vi "Get WhileLoop LoopTunnels.vi"(8 "error in":errorcluster, 11 "vi path":path=path "C:/Users/lubo/Documents/LabView/LabVIEW-Universal-Transcriptor/Test/Example Test 3.vi") -> (0 "error out":errorcluster, 2 "Tunnels Connected Wires Names":T2(array[cluster]), 3 "LoopTunnels with Terminals array":T3(array[cluster]))   [LabVIEW 2014]
doc: "Return array of clusters contains referencies to LoopTunnel for all WhileLoops. Each row in result array of cluster contain cluster with these items:\n - LoopTunnel ref. array\n - wires labels connected to InsideTerms[]"
uses:
  <vilib>/Utility/traverseref.llb/TRef TravTarget.ctl
  <vilib>/Utility/traverseref.llb/VI Scripting - Traverse.lvlib
panel:
  out "Tunnels Terminals Datatypes[][]":T1(array[cluster])
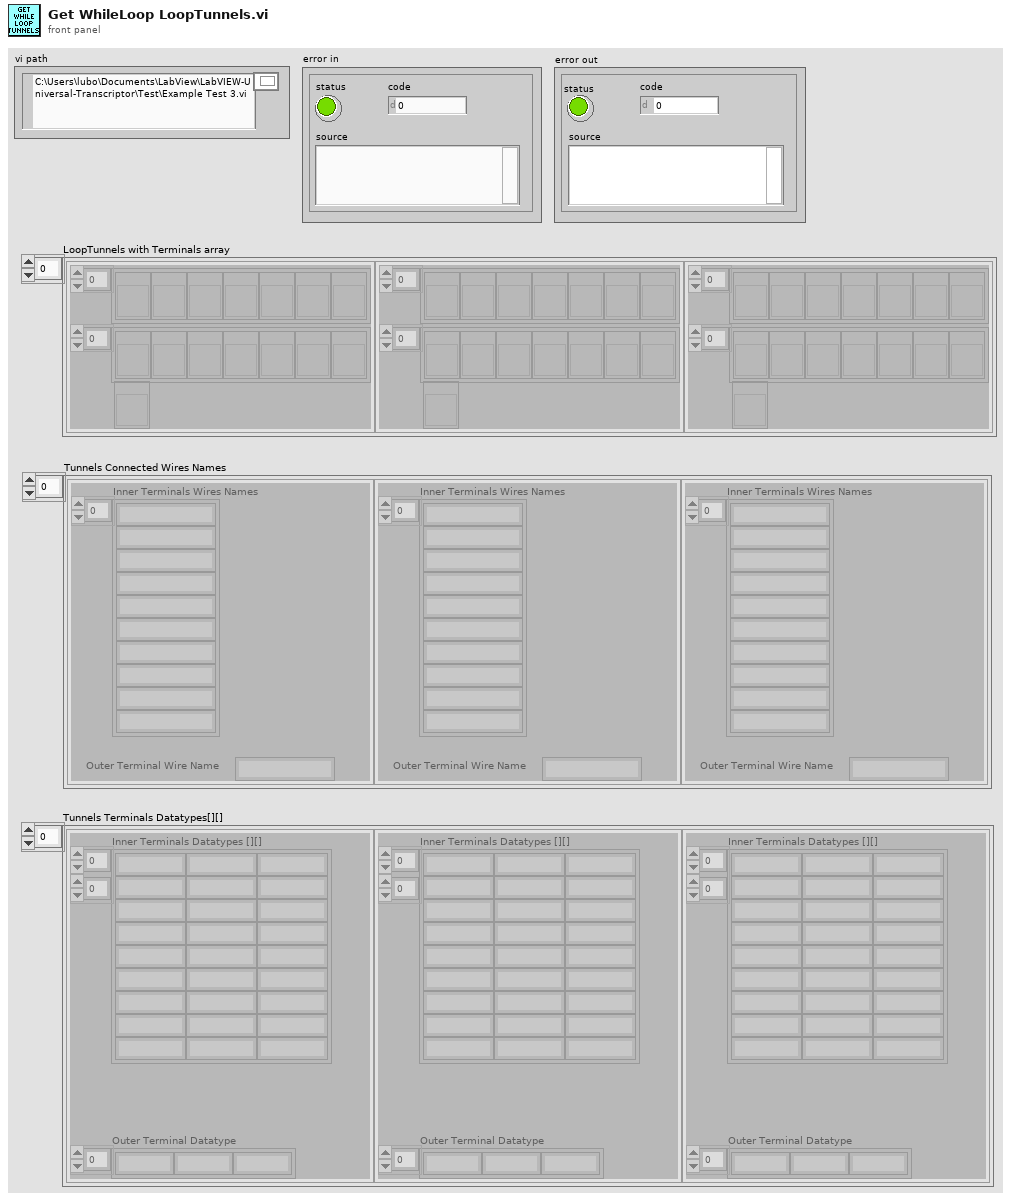
[diagram p1: front panel]
types:
  T1 = cluster{"Inner Terminals Datatypes [][]":string[][], "Outer Terminal Datatype":string[]}[]
  T2 = cluster{"Inner Terminals Wires Names":string[], "Outer Terminal Wire Name":string}[]
  T3 = cluster{refnum<vi>[], refnum<vi>[], refnum<vi>}[]
  T4 = typedef "TRef TravTarget.ctl" = enum16{"FP", "BD", "Other"}
  T5 = cluster{refnum<vi>[], "Inside Terminals[]":refnum<vi>[], "Outside Terminal":refnum<vi>}
  T6 = cluster{refnum<vi>[], "Inside Terminals[]":refnum<vi>[], "Outside Terminal":refnum<vi>}[]
  T7 = cluster{"Inner Terminals Wires Names":string[], "Outer Terminal Wire Name":string}
  T8 = cluster{"Inner Terminals Datatypes [][]":string[][], "Outer Terminal Datatype":string[]}
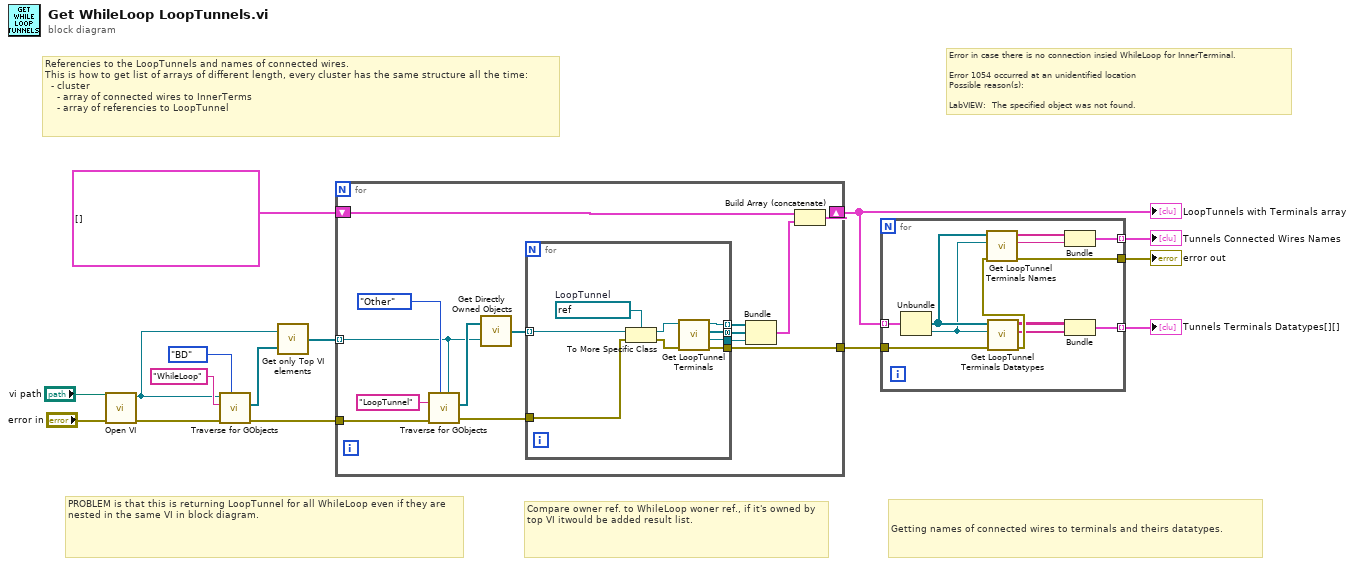
[diagram p0: block diagram]
diagram:
  # "Getting names of connected wires to terminals and theirs datatypes."
  # "Compare owner ref. to WhileLoop woner ref., if it's owned by top VI itwould be added result list."
  # "PROBLEM is that this is returning LoopTunnel for all WhileLoop even if they are nested in the same VI in block diagram."
  # "Error in case there is no connection insied WhileLoop for InnerTerminal.\n\nError 1054 occurred at an unidentified location\nPossible reason(s):\n\nLabVIEW:  The specified object was not found."
  # "Referencies to the LoopTunnels and names of connected wires.\nThis is how to get list of arrays of different length, every cluster has the same structure all the time:\n  - cluster\n    - array of connected wires to InnerTerms\n    - array of referencies to LoopTunnel"
  n1 = call "Open VI.vi"("error in"="error in", "vi path"="vi path") -> ("error out"=w12:errorcluster, "vi reference"=w8:refnum<vi>)  [unwired: 8 in]
  n2 = call <vilib>:"Traverse for GObjects.vi"("Traverse Target"=TRef_TravTarget."BD", "error in (no error)"=w12, "Class Name"="WhileLoop", "VI Refnum"=w8) -> ("error out"=w10:errorcluster, "References"=w7:refnum<vi>[])  [unwired: 4 in, 2 out]
  n3 = call "Get only Top VI elements.vi"("Ref. array in"=w7, "VI ref."=w8) -> ("Ref. array out"=w6:refnum<vi>[])
  n4 = for {
    tunnel: w10 -> [w29]
    tunnel: [w28] -> w4
    shift-right: [w23] -> w5
    shift-left: T3 [] -> [w27]
    tunnel: w6 -> [w20] mode=indexing
    n5 = call <vilib>:"Traverse for GObjects.vi"("Other Refnum"=w20, "Traverse Target"=TRef_TravTarget."Other", "error in (no error)"=w29, "Class Name"="LoopTunnel") -> ("error out"=w25:errorcluster, "References"=w22:refnum<vi>[])  [unwired: 4 in, 2 out]
    n6 = call "Get Directly Owned Objects.vi"("Top Object"=w20, "Nested Objects"=w22) -> ("Directly Owned Objects"=w21:refnum<vi>[])
    n7 = for {
      tunnel: w25 -> [w38]
      tunnel: [w37] -> w28
      tunnel: [w36] -> w19 mode=concatenating
      tunnel: w21 -> [w32] mode=indexing
      tunnel: [w31] -> w18
      tunnel: [w30] -> w17 mode=indexing
      w34 = refnum<vi> refnum  # LoopTunnel
      n8 = To More Specific Class(target class=w34, reference=w32, error in=w38) -> (specific class reference=w35:refnum<vi>, error out=w33:errorcluster)
      n9 = call "Get LoopTunnel Terminals.vi"("error in (no error)"=w33, "LoopTunnel in"=w35) -> ("error out"=w37:errorcluster, "Outside Terminal"=w31:refnum<vi>, "Inside Terminals[]"=w36:refnum<vi>[], "LoopTunnel out"=w30:refnum<vi>)  [unwired: 6 in]
    }
    n10 = Bundle(w17, "Inside Terminals[]"=w19, "Outside Terminal"=w18) -> (w16:T5)  [unwired: 1 in]
    n11 = Build Array (concatenate)(w27, w16) -> (w23:T6)
  }
  "LoopTunnels with Terminals array" <- w5
  n12 = for {
    tunnel: w5 -> [w50] mode=indexing
    tunnel: w4 -> [w45]
    tunnel: [w42] -> w2 mode=indexing
    tunnel: [w43] -> w3
    tunnel: [w41] -> w1 mode=indexing
    n13 = Unbundle(w50) -> (w47:refnum<vi>[], w46:refnum<vi>)  [unwired: 1 out]
    n14 = call "Get LoopTunnel Terminals Datatypes.vi"("Error In"=w45, "Outer Terminal"=w46, "Inner Terminals[]"=w47) -> ("Error Out"=w44:errorcluster, "Outer Terminal Datatype"=w39:string[], "Inner Terminals Datatypes [][]"=w40:string[][])  [unwired: 6 in]
    n15 = call "Get LoopTunnel Terminals Names.vi"("error in (no error)"=w44, "Outer Terminal"=w46, "Inside Terminals []"=w47) -> ("error out"=w43:errorcluster, "Outer Terminal Wire Name"=w49:string, "Inner Terminals Wires Names"=w48:string[])  [unwired: 6 in]
    n16 = Bundle("Inner Terminals Wires Names"=w48, "Outer Terminal Wire Name"=w49) -> (w42:T7)  [unwired: 1 in]
    n17 = Bundle("Inner Terminals Datatypes [][]"=w40, "Outer Terminal Datatype"=w39) -> (w41:T8)  [unwired: 1 in]
  }
  "error out" <- w3
  "Tunnels Connected Wires Names" <- w2
  "Tunnels Terminals Datatypes[][]" <- w1
